vi "Read Module NVMEM.vi"(8 "error in (no error)":errorcluster, 11 "SLSC Device":refnum<k21>) -> (0 "error out":errorcluster, 1 "slot number":u32, 2 "switches json":string, 3 "product name":string)   [LabVIEW 2017, in "SLSC Switch Examples.lvlib"]
uses:
  SLSC Switch Examples.lvlib
  <vilib>/SLSC/Initialize Session with Devices.vi
  <vilib>/SLSC/Close Session.vi
  <resource>/objmgr/slsc.rc
  <vilib>/SLSC/SLSC.lvlib
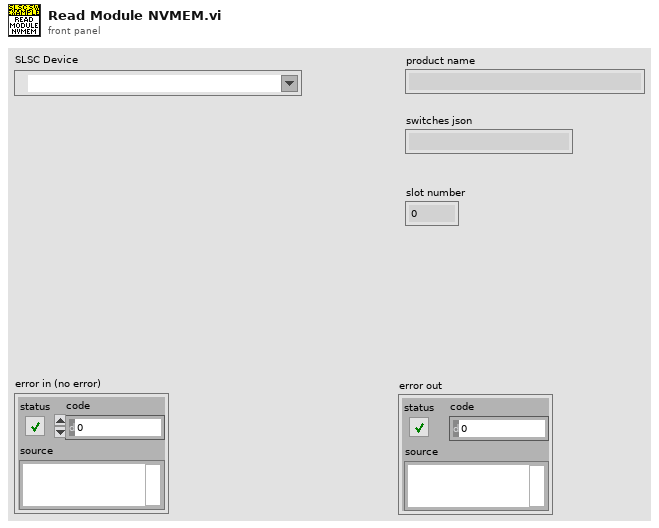
[diagram p1: front panel]
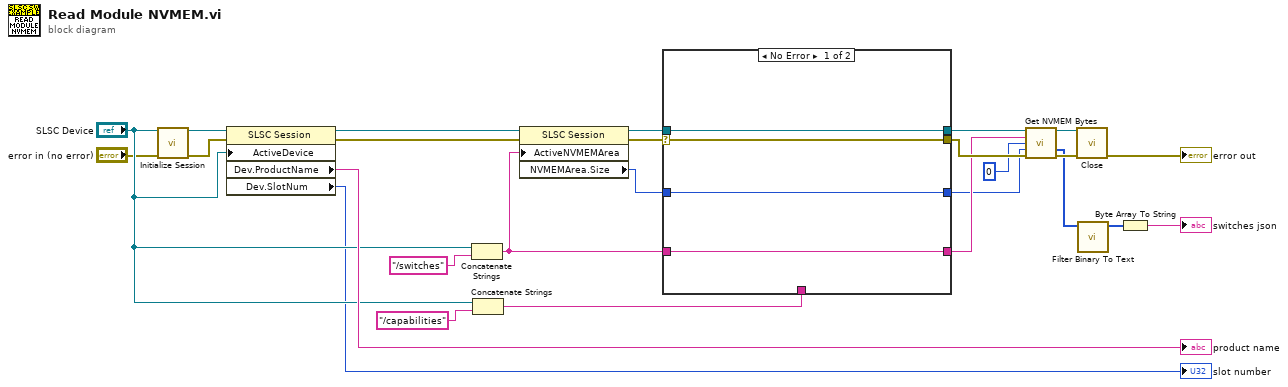
[diagram p0: block diagram]
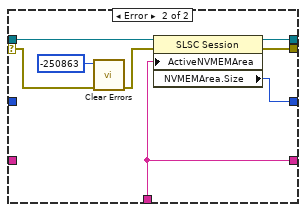
[diagram p2: hidden frame]
diagram:
  n1 = call-poly <vilib>:"Initialize Session.vi"("devices"="SLSC Device", "error in (no error)"="error in (no error)") -> ("session out"=w26:refnum<k21>, "error out"=w25:errorcluster)  [unwired: 12 in]
  n2 = property class="SLSC Session"(reference=w26, error in=w25, "ActiveDevice"="SLSC Device") -> (reference out=w23:refnum<k21>, error out=w20:errorcluster, "Dev.ProductName"=→"product name":string, "Dev.SlotNum"=→"slot number":u32)
  n3 = Concatenate Strings("SLSC Device", "/switches" ("string")) -> (w14:string)
  n4 = Concatenate Strings("SLSC Device", "/capabilities" ("string")) -> (w16:string)
  n5 = property class="SLSC Session"(reference=w23, error in=w20, "ActiveNVMEMArea"=w14) -> (reference out=w17:refnum<k21>, error out=w21:errorcluster, "NVMEMArea.Size"=w15:u32)
  n6 = case shown="No Error" w21 {
    selector: w21 -> [w27 w33]
    tunnel: w17 -> [w28 w38]
    tunnel: w16 -> [_ w36]
    tunnel: w15 -> [w29 _]
    tunnel: [w29 w37] -> w9
    tunnel: w14 -> [w30 _]
    tunnel: [w30 w36] -> w11
    tunnel: [w28 w35] -> w13
    tunnel: [w27 w34] -> w12
    frame No Error {
    }
    frame Error {
      n7 = call <vilib>:"Clear Errors.vi"("error in (no error)"=w33, "specific error code to clear (0: all)"=-250863) -> ("error out"=w32:errorcluster)  [unwired: 4 in, 1 out]
      n8 = property class="SLSC Session"(reference=w38, error in=w32, "ActiveNVMEMArea"=w36) -> (reference out=w35:refnum<k21>, error out=w34:errorcluster, "NVMEMArea.Size"=w37:u32)
    }
  }
  n9 = call <vilib>:"Get NVMEM Bytes.vi"("session in"=w13, "NVMEM area"=w11, "data address"=u32 0, "data size"=w9, "error in (no error)"=w12) -> ("session out"=w8:refnum<k21>, "data out"=w1:u8[], "error out"=w7:errorcluster)  [unwired: 6 in, 2 out]
  n10 = call-poly <vilib>:"Close.vi"("session in"=w8, "error in (no error)"=w7) -> ("error out"=→"error out":errorcluster)  [unwired: 13 in]
  n11 = call "Filter Binary To Text.vi"("Raw input"=w1) -> ("Filtered output"=w2:u8[])  [unwired: 10 in]
  n12 = Byte Array To String(unsigned byte array=w2) -> (string=→"switches json":string)
